vi "test.vi"() -> ()   [LabVIEW 2015]
panel:
  out "initialized array":dbl[](array[numeric])
  out "x-y":dbl
  in  "front margin (ns)":dbl format="%#_13g"
  in  "pi pulse (ns)":dbl format="%#_13g"
  in  "Array size":dbl format="%#_13g"
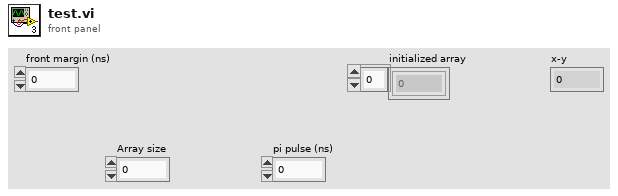
[diagram p1: front panel]
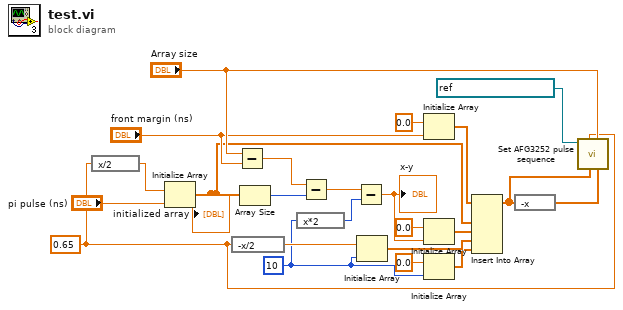
[diagram p0: block diagram]
diagram:
  w10 = 10 ("dimension size")
  w13 = 0.65 ("Gain (1 V)")
  n1 = expression code="x/2"(w13) -> (w22:dbl)
  n2 = Initialize Array(w22, "pi pulse (ns)") -> (w15:dbl[])
  "initialized array" <- w15
  n3 = expression code="-x/2"(w13) -> (w12:dbl)
  n4 = Subtract(x="Array size", y="front margin (ns)") -> (x-y=w16:dbl)
  n5 = Array Size(array=w15) -> (size(s)=w14:i32)
  n6 = expression code="x*2"(w10) -> (w8:i32)
  n7 = Subtract(x=w16, y=w14) -> (x-y=w9:dbl)
  n8 = Subtract(x=w9, y=w8) -> (x-y=w7:dbl)
  "x-y" <- w7
  n9 = Initialize Array(w12, w10) -> (w4:dbl[])
  n10 = Initialize Array(0.0 ("element"), "front margin (ns)") -> (w19:dbl[])
  n11 = Initialize Array(0.0 ("element"), w7) -> (w5:dbl[])
  n12 = Initialize Array(0.0 ("element"), w10) -> (w3:dbl[])
  n13 = Insert Into Array(array=w19, new element #1=w15, new element #2=w5, new element #3=w4, new element #4=w3) -> (w2:dbl[])  [unwired: 1 in]
  n14 = expression code="-x"(w2) -> (w1:dbl[])
  n15 = call "Set AFG3252 pulse sequence.vi"("Channel 2"=w1, "Array size"="Array size", "Channel 1"=w2, "Gain (1 V)"=w13, "VISA resource name"=refnum<visa-resource-name> "GPIB0::16::INSTR") -> ()  [unwired: 7 in]
